vi "MoveTrackShow_old.vi"(7 "Cursor Position":T1={"Left"=400, "Top"=400, "Right"=600, "Bottom"=600}, 9 "ZoomInteger:All Elements":cluster{"X":i32, "Y":i32}, 10 "Image Area:Size:All Elements":cluster{"Width":u32, "Height":u32}, 11 "Image Center Position:All Elements":cluster{"X":u32, "Y":u32}) -> (3 "Centre Position":cluster{"X":u32, "Y":u32})   [LabVIEW 2014]
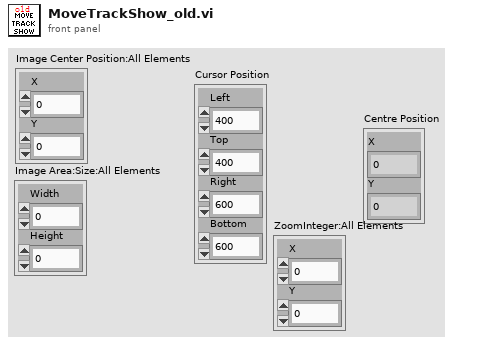
[diagram p1: front panel]
types:
  T1 = cluster{"Left":i32, "Top":i32, "Right":i32, "Bottom":i32}
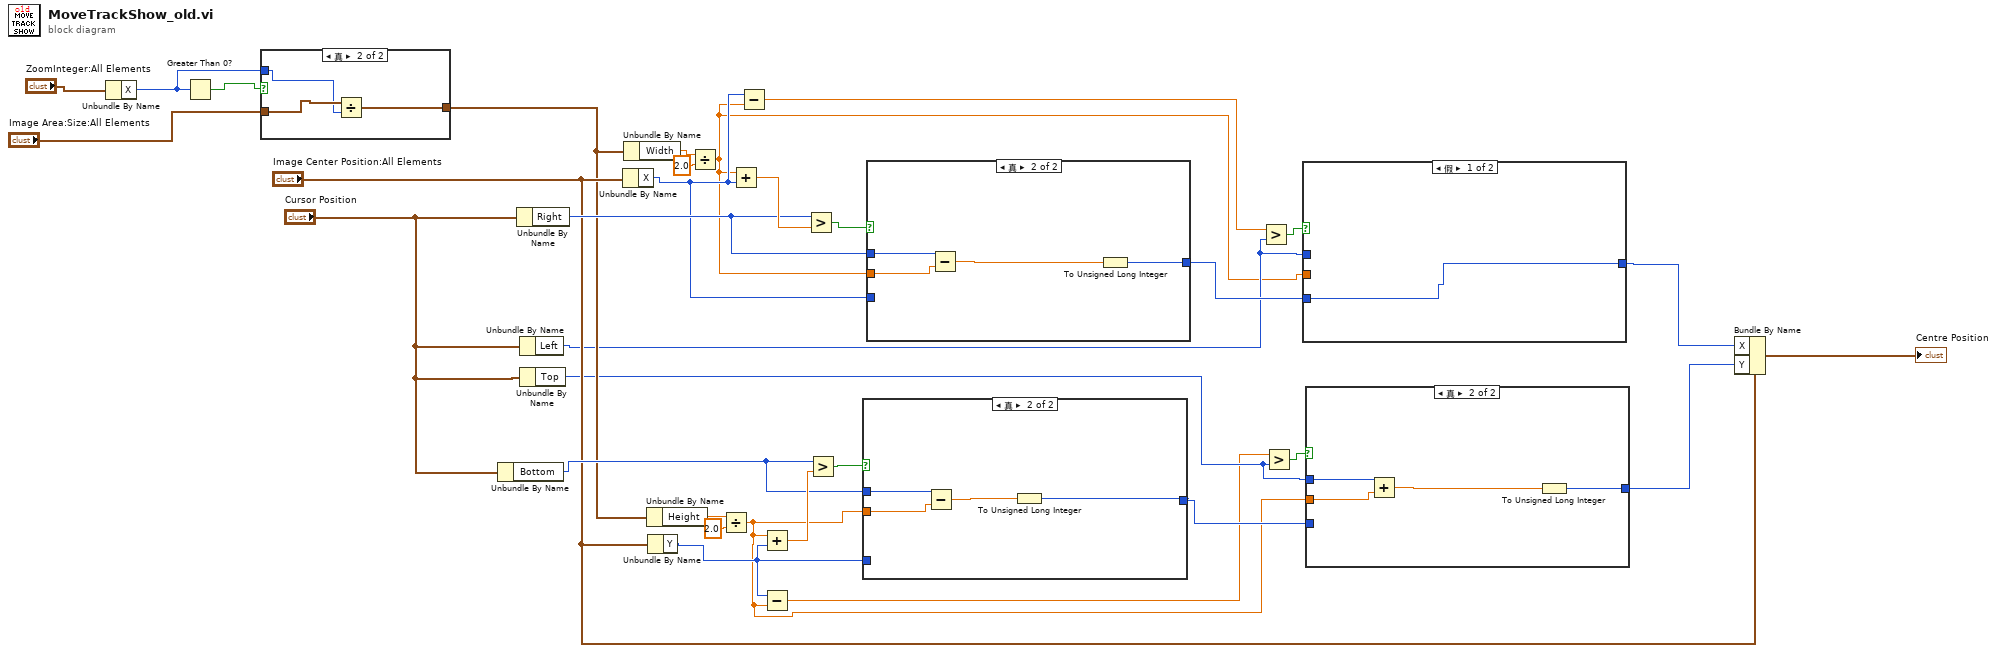
[diagram p0: block diagram]
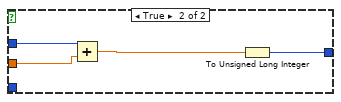
[diagram p3: hidden frame]
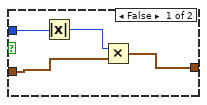
[diagram p4: hidden frame]
diagram:
  n1 = Unbundle By Name("ZoomInteger:All Elements") -> ("X"=w18:i32)
  n2 = Greater Than 0?(x=w18) -> (x > 0?=w19:bool)
  n3 = case shown="真" w19 {
    tunnel: "Image Area:Size:All Elements" -> [w34 w39]
    tunnel: w18 -> [w36 w38]
    tunnel: [w33 w37] -> w17
    frame False {
      n4 = Absolute Value(x=w36) -> (abs(x)=w35:i32)
      n5 = Multiply(x=w35, y=w34) -> (x*y=w33:cluster{"Width":u32, "Height":u32})
    }
    frame True {
      n6 = Divide(x=w39, y=w38) -> (x/y=w37:cluster{"Width":dbl, "Height":dbl})
    }
  }
  n7 = Unbundle By Name("Cursor Position") -> ("Bottom"=w23:i32)
  n8 = Unbundle By Name("Cursor Position") -> ("Right"=w28:i32)
  n9 = Unbundle By Name("Cursor Position") -> ("Left"=w11:i32)
  n10 = Unbundle By Name("Cursor Position") -> ("Top"=w7:i32)
  n11 = Unbundle By Name("Image Center Position:All Elements") -> ("X"=w14:u32)
  n12 = Unbundle By Name(w17) -> ("Width"=w32:dbl)
  n13 = Unbundle By Name(w17) -> ("Height"=w26:dbl)
  n14 = Unbundle By Name("Image Center Position:All Elements") -> ("Y"=w6:u32)
  n15 = Divide(x=w32, y=2.0) -> (x/y=w2:dbl)
  n16 = Divide(x=w26, y=2.0) -> (x/y=w3:dbl)
  n17 = Add(x=w2, y=w14) -> (x+y=w30:dbl)
  n18 = Subtract(x=w14, y=w2) -> (x-y=w1:dbl)
  n19 = Add(x=w3, y=w6) -> (x+y=w25:dbl)
  n20 = Subtract(x=w6, y=w3) -> (x-y=w5:dbl)
  n21 = Greater?(x=w28, y=w30) -> (0:w29:bool)
  n22 = Greater?(x=w23, y=w25) -> (0:w24:bool)
  n23 = case shown="真" w24 {
    tunnel: w23 -> [_ w44]
    tunnel: w3 -> [_ w43]
    tunnel: w6 -> [w40 _]
    tunnel: [w40 w41] -> w8
    frame False {
    }
    frame True {
      n24 = Subtract(x=w44, y=w43) -> (x-y=w42:dbl)
      n25 = To Unsigned Long Integer(number=w42) -> (unsigned 32bit integer=w41:u32)
    }
  }
  n26 = case shown="真" w29 {
    tunnel: w28 -> [_ w49]
    tunnel: w2 -> [_ w48]
    tunnel: w14 -> [w45 _]
    tunnel: [w45 w46] -> w15
    frame False {
    }
    frame True {
      n27 = Subtract(x=w49, y=w48) -> (x-y=w47:dbl)
      n28 = To Unsigned Long Integer(number=w47) -> (unsigned 32bit integer=w46:u32)
    }
  }
  n29 = Greater?(x=w1, y=w11) -> (0:w12:bool)
  n30 = Greater?(x=w5, y=w7) -> (0:w9:bool)
  n31 = case shown="假" w12 {
    tunnel: w11 -> [_ w54]
    tunnel: w2 -> [_ w53]
    tunnel: w15 -> [w50 _]
    tunnel: [w50 w51] -> w10
    frame False {
    }
    frame True {
      n32 = Add(x=w54, y=w53) -> (x+y=w52:dbl)
      n33 = To Unsigned Long Integer(number=w52) -> (unsigned 32bit integer=w51:u32)
    }
  }
  n34 = case shown="真" w9 {
    tunnel: w7 -> [_ w59]
    tunnel: w3 -> [_ w58]
    tunnel: w8 -> [w55 _]
    tunnel: [w55 w56] -> w4
    frame False {
    }
    frame True {
      n35 = Add(x=w59, y=w58) -> (x+y=w57:dbl)
      n36 = To Unsigned Long Integer(number=w57) -> (unsigned 32bit integer=w56:u32)
    }
  }
  n37 = Bundle By Name(cluster="Image Center Position:All Elements", "X"=w10, "Y"=w4) -> (→"Centre Position":cluster{"X":u32, "Y":u32})
